vi "Calc_R.vi"(2 "He_spectrum":dbl[](array[numeric]), 3 "Zero_spectrum":dbl[](array[numeric]), 4 "Density zero":dbl, 5 "Rayleigh R":dbl[](array[numeric]), 6 "Rayleigh zero":dbl[](array[numeric]), 8 "Density R":dbl, 12 "Length_cm":dbl) -> (20 "Reflectivity":dbl[](array[numeric]))   [LabVIEW 2025]
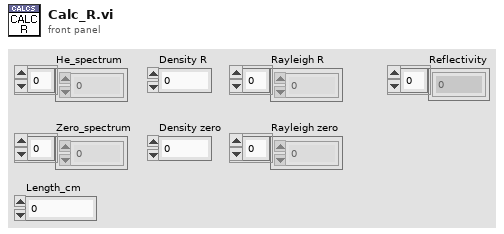
[diagram p1: front panel]
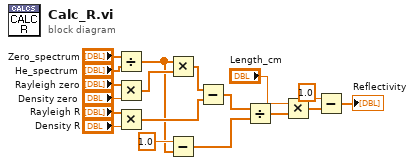
[diagram p0: block diagram]
diagram:
  n1 = Divide(x="Zero_spectrum", y="He_spectrum") -> (x/y=w4:dbl[])
  n2 = Multiply(x="Rayleigh zero", y="Density zero") -> (x*y=w8:dbl[])
  n3 = Multiply(x="Rayleigh R", y="Density R") -> (x*y=w6:dbl[])
  n4 = Multiply(x=w4, y=w8) -> (x*y=w7:dbl[])
  n5 = Subtract(x=1.0, y=w4) -> (x-y=w2:dbl[])
  n6 = Subtract(x=w7, y=w6) -> (x-y=w3:dbl[])
  n7 = Divide(x=w3, y=w2) -> (x/y=w1:dbl[])
  n8 = Multiply(x="Length_cm", y=w1) -> (x*y=w13:dbl[])
  n9 = Subtract(x=1.0, y=w13) -> (x-y=→"Reflectivity":dbl[])
